vi "GEN_ResetTimer.vi"(8 "error in (no error)":errorcluster, 9 "Data_In":T3={"Value"=0.0, "GUI Data Cluster"={"SBR"=0}, "Timing"={"Last Operation"=0.0, "Stop @ T"=FALSE, "Delta T Log"=FALSE, "End T"=0.0, "Delta T"=0.0, "Last Temp"=0.0}, "Measurements"=[], "Hardware"={"VNA TCP Con"=refnum, "VNA TCP Port"=5025, "Global T VAR"="", "Global B VAR"=""}, "Operation"={"Operation Mode"=enum."Logging", "Status"="", "NewLog?"=FALSE}} {"GUI Data Cluster"."SBR" format="%08b"}, 10 "Cluster IN":T1={"General"={"Config.ini"=path "", "Default Logging Path"=path ""}, "Hardware"={"Measure Rate (1/s)"=0, "HP DMM VISA"="", "LS 335 VISA"="", "HP DM"={"Range"=enum."Autorange", "Autozero"=FALSE, "Display"=enum."3 1/2 Digit", "Blank LCD"=FALSE}}, "Operation"={"Operation Mode"=enum."Idle-Off", "Status"="", "NewLog?"=FALSE, "OvenWarn"=FALSE}}) -> (0 "error out":errorcluster, 1 "Data_In 2":T3={"Value"=0.0, "GUI Data Cluster"={"SBR"=0}, "Timing"={"Last Operation"=0.0, "Stop @ T"=FALSE, "Delta T Log"=FALSE, "End T"=0.0, "Delta T"=0.0, "Last Temp"=0.0}, "Measurements"=[], "Hardware"={"VNA TCP Con"=refnum, "VNA TCP Port"=5025, "Global T VAR"="", "Global B VAR"=""}, "Operation"={"Operation Mode"=enum."Logging", "Status"="", "NewLog?"=FALSE}} {"GUI Data Cluster"."SBR" format="%08b"}, 2 "Cluster OUT":T1={"General"={"Config.ini"=path "", "Default Logging Path"=path ""}, "Hardware"={"Measure Rate (1/s)"=0, "HP DMM VISA"="", "LS 335 VISA"="", "HP DM"={"Range"=enum."Autorange", "Autozero"=FALSE, "Display"=enum."3 1/2 Digit", "Blank LCD"=FALSE}}, "Operation"={"Operation Mode"=enum."Idle-Off", "Status"="", "NewLog?"=FALSE, "OvenWarn"=FALSE}}, 4 "TimeStamp":timestamp)   [LabVIEW 2021]
uses:
  Data_Cluster.ctl
  Measurement_Cluster.ctl
  Mode_Enum.ctl
  Config_Cluster.ctl
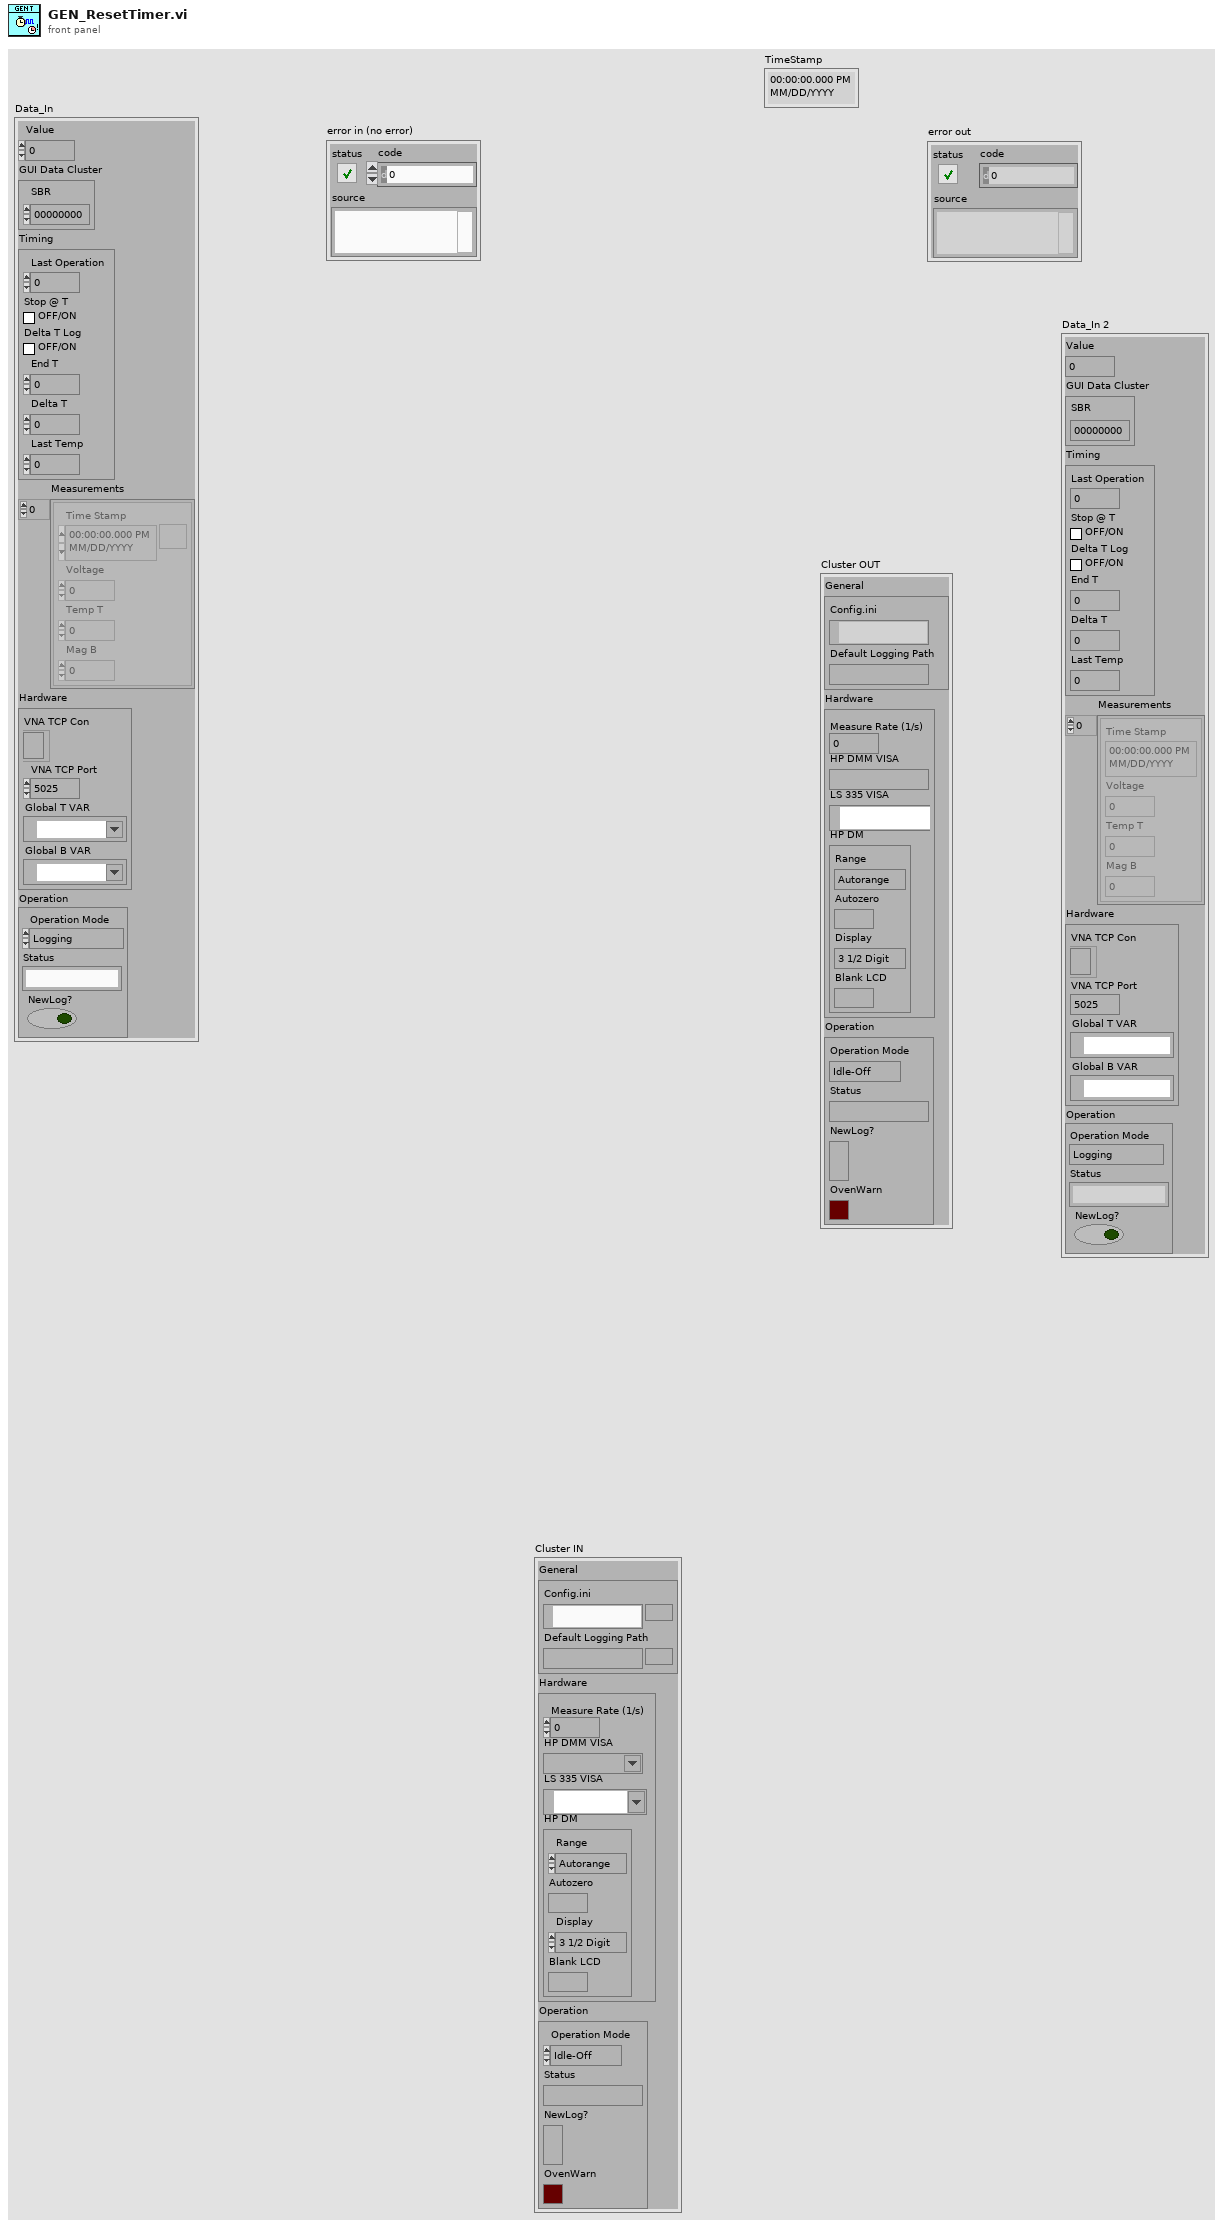
[diagram p1: front panel]
types:
  T1 = typedef "Config_Cluster.ctl" = cluster{"General":cluster{"Config.ini":path, "Default Logging Path":path}, "Hardware":cluster{"Measure Rate (1/s)":i32, "HP DMM VISA":refnum<visa-resource-name>, "LS 335 VISA":refnum<visa-resource-name>, "HP DM":cluster{"Range":enum16{"Autorange", "30mV", "300mV", "3V", "30V"}, "Autozero":bool, "Display":enum16{"3 1/2 Digit", "4 1/2 Digit", "5 1/2 Digit"}, "Blank LCD":bool}}, "Operation":cluster{"Operation Mode":T2, "Status":string, "NewLog?":bool, "OvenWarn":bool}}
  T2 = typedef "Mode_Enum.ctl" = enum16{"OvenNRDY", "Logging", "Idle-Off", "Idle"}
  T3 = typedef "Data_Cluster.ctl" = cluster{"Value":dbl, "GUI Data Cluster":cluster{"SBR":u16}, "Timing":cluster{"Last Operation":dbl, "Stop @ T":bool, "Delta T Log":bool, "End T":dbl, "Delta T":dbl, "Last Temp":dbl}, "Measurements":T4[], "Hardware":cluster{"VNA TCP Con":refnum<k5>, "VNA TCP Port":i32, "Global T VAR":refnum<k21>, "Global B VAR":refnum<k21>}, "Operation":cluster{"Operation Mode":T2, "Status":string, "NewLog?":bool}}
  T4 = typedef "Measurement_Cluster.ctl" = cluster{"Time Stamp":timestamp, "Voltage":dbl, "Temp T":dbl, "Mag B":dbl}
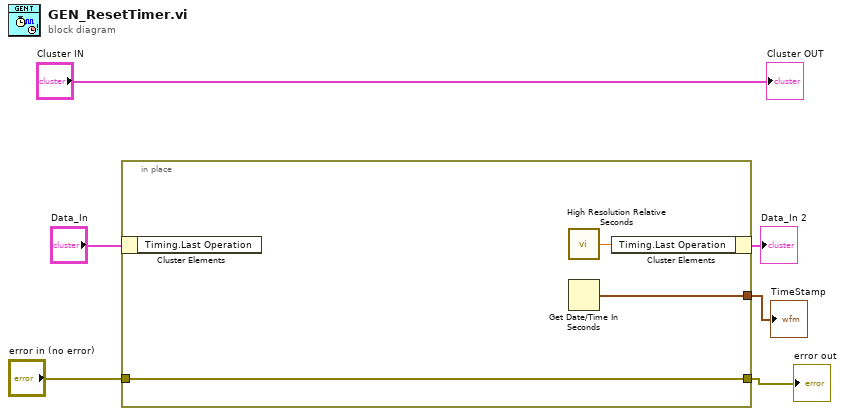
[diagram p0: block diagram]
diagram:
  n1 = in-place {
    in-place-border: [w8] -> w4
    in-place-border: "error in (no error)" -> [w7]
    in-place-border: [w7] -> w2
    n2 = in-place-cluster #1("Data_In") -> ()  [unwired: 1 out]
    n3 = call <vilib>:"High Resolution Relative Seconds.vi"() -> ("relative seconds"=w9:dbl)
    n4 = Get Date/Time In Seconds() -> (seconds since 1Jan1904=w8:timestamp)
    n5 = in-place-cluster #1("Timing.Last Operation"=w9) -> (→"Data_In 2":T3)
  }
  "TimeStamp" <- w4
  "error out" <- w2
  "Cluster OUT" <- "Cluster IN"
